vi "get_term_index.vi"(8 "error in (no error)":errorcluster, 11 "Last Function Ref In":refnum<vi>) -> (0 "error out":errorcluster, 2 "Term Index":i32, 3 "Last Function Ref Out":refnum<vi>)   [LabVIEW 2018]
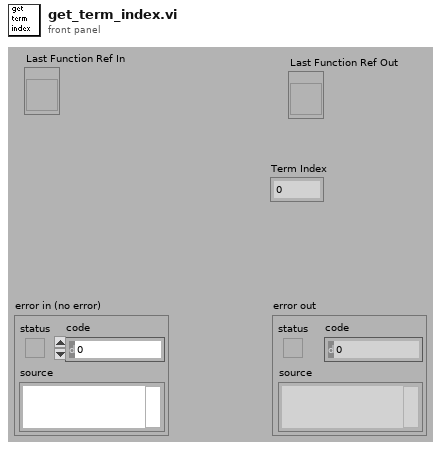
[diagram p1: front panel]
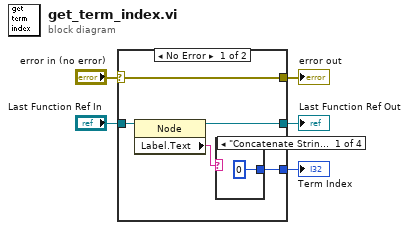
[diagram p0: block diagram]
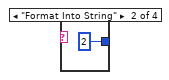
[diagram p2: hidden frame]
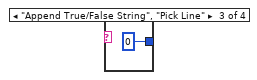
[diagram p3: hidden frame]
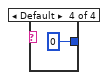
[diagram p4: hidden frame]
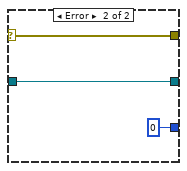
[diagram p5: hidden frame]
diagram:
  n1 = case shown="No Error" "error in (no error)" {
    selector: "error in (no error)" -> [w6 w17]
    tunnel: "Last Function Ref In" -> [w10 w16]
    tunnel: [w8 0 ("index")] -> w4
    tunnel: [w7 w16] -> w3
    tunnel: [w6 w17] -> w1
    frame No Error {
      n2 = property class="Node"(reference=w10) -> (reference out=w7:refnum<vi>, "Label.Text"=w9:string)  [unwired: 1 in, 1 out]
      n3 = case shown="\"Concatenate Strings\"" w9 {
        tunnel: [0 ("index") 2 ("index") 0 ("index") 0 ("index")] -> w8
        frame "Concatenate Strings" {
        }
        frame "Format Into String" {
        }
        frame "Append True/False String", "Pick Line" {
        }
        frame Default {
        }
      }
    }
    frame Error {
    }
  }
  "Term Index" <- w4
  "Last Function Ref Out" <- w3
  "error out" <- w1
